vi "GUI.vi"() -> ()   [LabVIEW 2020]
uses:
  <vilib>/Instr/_visa.llb/VISA Configure Serial Port (Instr).vi
panel:
  out "Device name":string
  in  "VISA resource name":refnum<visa-resource-name>="COM6"
  in  "Shutter":bool
  in  "Power (%)":dbl(slide)=100.0 scale=0.0..100.0
  out "Emitting:":bool=TRUE
  in  "stop":bool
  # "Analog control AOMs Salix"
  # "515 nm"
  # "561 nm"
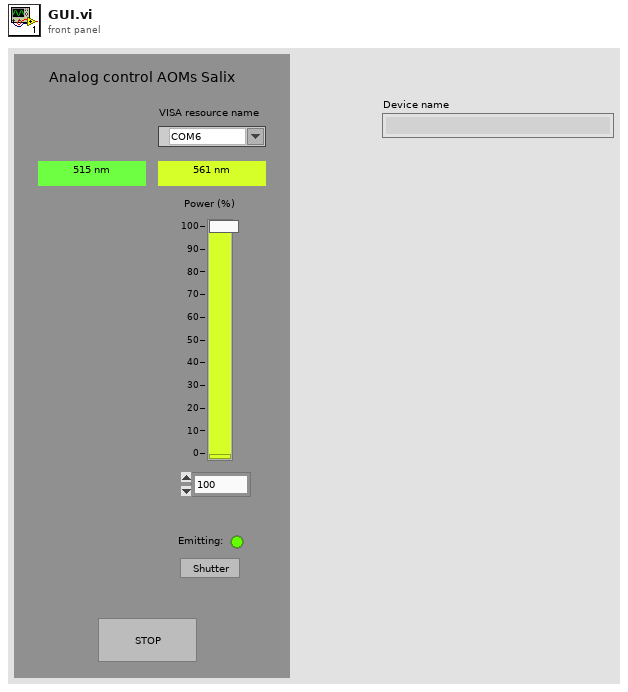
[diagram p1: front panel]
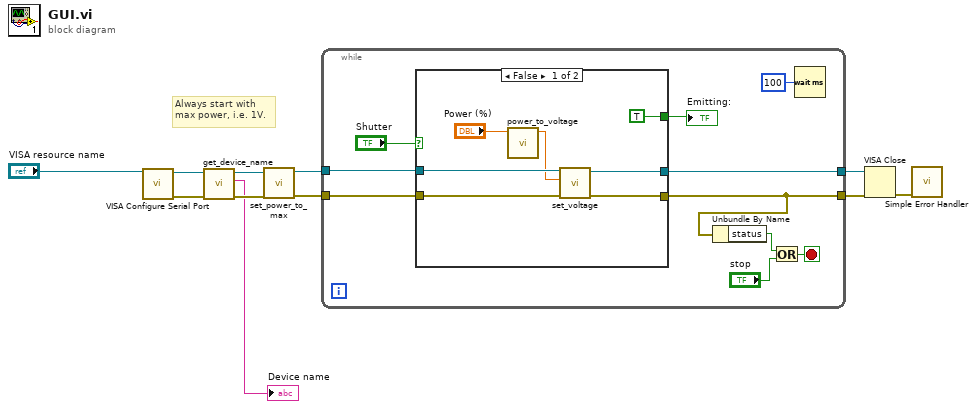
[diagram p0: block diagram]
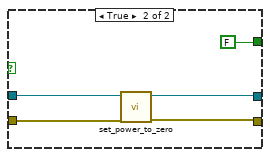
[diagram p2: hidden frame]
diagram:
  # "Always start with\nmax power, i.e. 1V."
  n1 = call-poly "VISA Configure Serial Port"("VISA resource name"="VISA resource name") -> ("VISA resource name out"=w2:refnum<visa-resource-name>, "error out"=w3:errorcluster)  [unwired: 9 in, 4 out]
  n2 = call "get_device_name.vi"("error in"=w3, "VISA resource name in"=w2) -> ("error out"=w4:errorcluster, "Device name"=→"Device name":string, "VISA resource name out"=w5:refnum<visa-resource-name>)  [unwired: 7 in]
  n3 = call "set_power_to_max.vi"("error in"=w4, "VISA resource name"=w5) -> ("error out"=w10:errorcluster, "VISA resource name out"=w11:refnum<visa-resource-name>)  [unwired: 8 in]
  n4 = while {
    tunnel: w11 -> [w20]
    tunnel: w10 -> [w19]
    tunnel: [w17] -> w7
    tunnel: [w13] -> w6
    stop <- w21 stop-if-true
    n5 = case shown="False" "Shutter" {
      tunnel: w20 -> [w24 w32]
      tunnel: w19 -> [w26 w31]
      tunnel: [w25 w30] -> w17
      tunnel: [TRUE ("Boolean") FALSE ("Boolean")] -> w15
      tunnel: [w23 w29] -> w13
      frame False {
        n6 = call "power_to_voltage.vi"("Power"="Power (%)") -> ("Voltage"=w22:dbl)  [unwired: 10 in]
        n7 = call "set_voltage.vi"("error in"=w26, "voltage"=w22, "VISA resource name"=w24) -> ("error out"=w25:errorcluster, "VISA resource name out"=w23:refnum<visa-resource-name>)  [unwired: 6 in, 1 out]
      }
      frame True {
        n8 = call "set_power_to_zero.vi"("error in"=w31, "VISA resource name"=w32) -> ("error out"=w30:errorcluster, "VISA resource name out"=w29:refnum<visa-resource-name>)  [unwired: 8 in]
      }
    }
    "Emitting:" <- w15
    n9 = Unbundle By Name(w17) -> ("status"=w18:bool)
    n10 = Or(x=w18, y="stop") -> (x .or. y?=w21:bool)
    n11 = Wait (ms)(milliseconds to wait=u32 100) -> ()  [unwired: 1 out]
  }
  n12 = VISA Close(VISA resource name=w6, error in (no error)=w7) -> (error out=w8:errorcluster)
  n13 = call <vilib>:"Simple Error Handler.vi"("error in (no error)"=w8) -> ()  [unwired: 1 in, 8 out]
